vi "SubVI_TurnRight_Auto.vi"(7 "PIDF":dbl[](array[numeric]), 8 "angular Speed":dbl=1000.0, 9 "Degrees to target":dbl) -> ()   [LabVIEW 2017]
uses:
  <vilib>/Rock Robotics/WPI/ThirdParty/Sensors/navX/_TypeDefs/Z900_navX_ActionTypeDef.ctl
  <vilib>/Rock Robotics/WPI/ThirdParty/Sensors/navX/_TypeDefs/FRIC_navX_DeviceNumbersTypeDef.ctl
  <vilib>/Rock Robotics/WPI/ThirdParty/Phoenix-LabVIEW/Motor Controller/Controls/CTRE_Phoenix_MotorControl_ControlMode.ctl
panel:
  out "Yaw":dbl
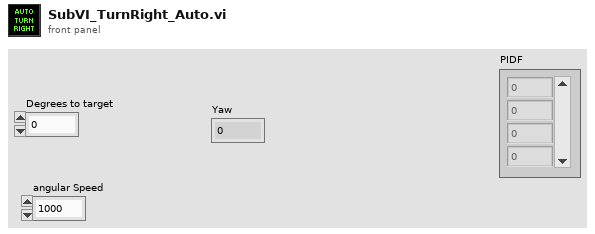
[diagram p1: front panel]
types:
  T1 = typedef "FRIC_navX_DeviceNumbersTypeDef.ctl" = enum16{"Dev0", "Dev1", "Dev2", "Dev3"}
  T2 = typedef "Z900_navX_ActionTypeDef.ctl" = enum16{"None", "Halt", "Normal Read", "Update Serial Protocol", "Update Rate Htz", "Zero-Yaw", "Zero-Displacement", "Zero-Velocity"}
  T3 = typedef "WPI_MotorControlDeviceRef.ctl" = cluster{"DeviceStatus":errorcluster, "Type":T4, "PWM":cluster{"PWM Channel":T5, "DeadBand":T6}, "CAN":cluster{"Device Number":u8, "SetOutput VI Ref":variant, "GetOutput VI Ref":variant, "Enable VI Ref":variant, "Disable VI Ref":variant, "Data":variant}, "Invert":bool, "DIO PWM":cluster{"PWM \"Enable\" Channel":T5, "DIOChannel":T7, "PWM Rate":dbl}}
  T4 = typedef "WPI_MotorControlType.ctl" = enum16{"PWM", "CAN", "DIO PWM"}
  T5 = typedef "FPGA_DIOPWMChannel.ctl" = enum8{"PWM 0", "PWM 1", "PWM 2", "PWM 3", "PWM 4", "PWM 5", "PWM 6", "PWM 7", "PWM 8", "PWM 9", "PWM MXP 0", "PWM MXP 1", "PWM MXP 2", "PWM MXP 3", "PWM MXP 4", "PWM MXP 5", "PWM MXP 6", "PWM MXP 7", "PWM MXP 8", "PWM MXP 9", "Invalid"}
  T6 = typedef "WPI_PWMDeadband.ctl" = cluster{"Name":string, "maxPositivePwm":i32, "minPositivePwm":i32, "centerPwm":i32, "maxNegativePwm":i32, "minNegativePwm":i32, "angularRange":u16}
  T7 = typedef "FPGA_DIOChannel.ctl" = enum8{"DIO 0", "DIO 1", "DIO 2", "DIO 3", "DIO 4", "DIO 5", "DIO 6", "DIO 7", "DIO 8", "DIO 9", "DIO MXP 0", "DIO MXP 1", "DIO MXP 2", "DIO MXP 3", "DIO MXP 4", "DIO MXP 5", "DIO MXP 6", "DIO MXP 7", "DIO MXP 8", "DIO MXP 9", "DIO MXP 10", "DIO MXP 11", "DIO MXP 12", "DIO MXP 13", "DIO MXP 14", "DIO MXP 15", "SPI Port CS1", "SPI Port CS2", "SPI Port CS3", "SPI Port MISO", "SPI Port MOSI", "Invalid"}
  T8 = cluster{"Yaw":dbl, "Roll":dbl, "Pitch":dbl, "Heading":dbl, "Fused Heading":dbl}
  T9 = typedef "CTRE_Phoenix_MotorControl_ControlMode.ctl" = u16
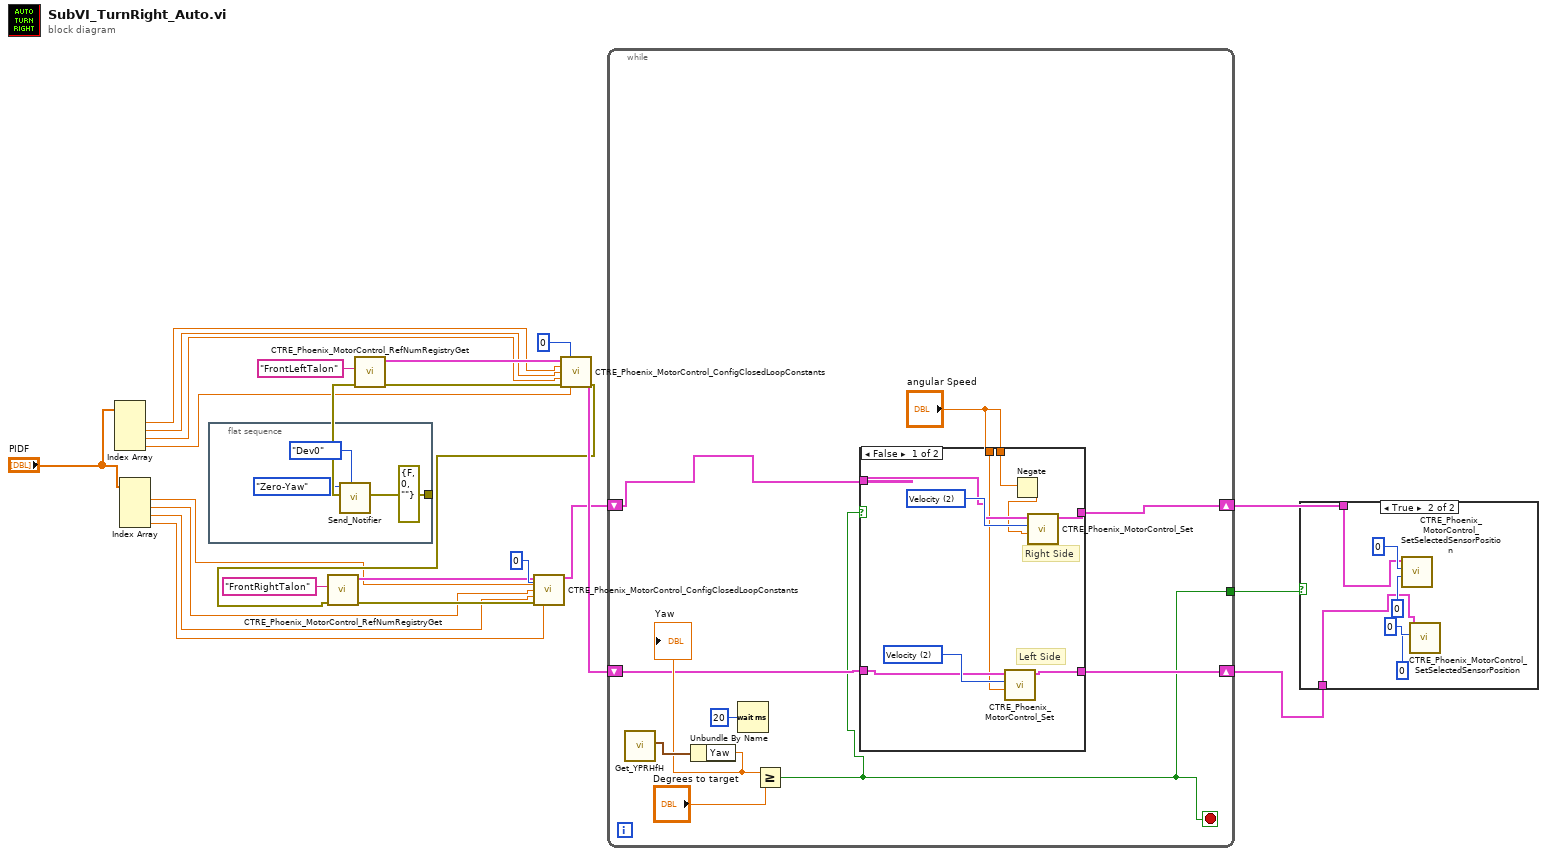
[diagram p0: block diagram]
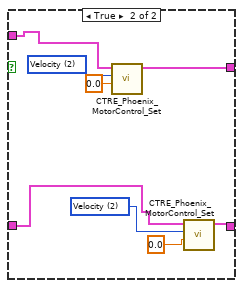
[diagram p3: hidden frame]
diagram:
  n1 = Index Array(array="PIDF") -> (element #1=w11:dbl, element #2=w10:dbl, element #3=w9:dbl, element #4=w8:dbl)  [unwired: 4 in]
  n2 = Index Array(array="PIDF") -> (element #1=w7:dbl, element #2=w6:dbl, element #3=w5:dbl, element #4=w4:dbl)  [unwired: 4 in]
  n3 = flat-sequence {
    tunnel: [errorcluster {"status"=FALSE, "code"=0, "source"=""} ("error constant")] -> w13
    frame #0 {
      n4 = call <vilib>:"Send_Notifier.vi"("Device Number"=FRIC_navX_DeviceNumbersTypeDef."Dev0", "navX Action"=Z900_navX_ActionTypeDef."Zero-Yaw") -> ()  [unwired: 10 in]
    }
  }
  n5 = call <vilib>:"CTRE_Phoenix_MotorControl_RefNumRegistryGet.vi"("error in (no error)"=w13, "refnum name"="FrontLeftTalon") -> ("error out"=w17:errorcluster, "PhoenixMotorControlDevRef"=w18:T3)  [unwired: 8 in]
  n6 = call <vilib>:"CTRE_Phoenix_MotorControl_ConfigClosedLoopConstants.vi"("PhoenixMotorControlDevRef"=w18, "slotIdx"=0, "P"=w11, "I"=w10, "D"=w9, "error in (no error)"=w17, "F"=w8) -> ("PhoenixMotorControlDevRef"=w23:T3, "error out"=w14:errorcluster)  [unwired: 7 in]
  n7 = call <vilib>:"CTRE_Phoenix_MotorControl_RefNumRegistryGet.vi"("error in (no error)"=w14, "refnum name"="FrontRightTalon") -> ("error out"=w15:errorcluster, "PhoenixMotorControlDevRef"=w16:T3)  [unwired: 8 in]
  n8 = call <vilib>:"CTRE_Phoenix_MotorControl_ConfigClosedLoopConstants.vi"("PhoenixMotorControlDevRef"=w16, "slotIdx"=0, "P"=w7, "I"=w6, "D"=w5, "error in (no error)"=w15, "F"=w4) -> ("PhoenixMotorControlDevRef"=w19:T3)  [unwired: 7 in, 1 out]
  n9 = while {
    shift-right: [w31] -> w2
    shift-left: w23 -> [w32]
    shift-right: [w37] -> w3
    shift-left: w19 -> [w35]
    tunnel: [w28] -> w1
    stop <- w28 stop-if-true
    n10 = call <vilib>:"Get_YPRHfH.vi"() -> ("YRPHfH"=w34:T8)  [unwired: 11 in]
    n11 = Unbundle By Name(w34) -> ("Yaw"=w33:dbl)
    "Yaw" <- w33
    n12 = Wait (ms)(milliseconds to wait=u32 20) -> ()  [unwired: 1 out]
    n13 = Greater Or Equal?(x=w33, y="Degrees to target") -> (x >= y?=w28:bool)
    n14 = case shown="False" w28 {
      tunnel: [w45 w52] -> w37
      tunnel: w35 -> [w44 w51]
      tunnel: w32 -> [w42 w49]
      tunnel: [w41 w47] -> w31
      tunnel: "angular Speed" -> [w39 _]
      tunnel: "angular Speed" -> [w40 _]
      frame False {
        w43 = T9 2 items=["PercentOutput"=0, "Position"=1, "Velocity"=2, "Current"=3, "Follower"=5, "MotionProfile"=6, "MotionMagic"=7, "MotionMagicArc"=8, "MotionProfileArc"=10, "Disabled"=15] ("Control Mode")
        w46 = T9 2 items=["PercentOutput"=0, "Position"=1, "Velocity"=2, "Current"=3, "Follower"=5, "MotionProfile"=6, "MotionMagic"=7, "MotionMagicArc"=8, "MotionProfileArc"=10, "Disabled"=15] ("Control Mode")
        # "Right Side"
        # "Left Side"
        n15 = call <vilib>:"CTRE_Phoenix_MotorControl_Set.vi"("Output"=w40, "Control Mode"=w43, "PhoenixMotorControlDevRef"=w42) -> ("PhoenixMotorControlDevRef"=w41:T3)  [unwired: 7 in, 1 out]
        n16 = Negate(x=w39) -> (-x=w38:dbl)
        n17 = call <vilib>:"CTRE_Phoenix_MotorControl_Set.vi"("Output"=w38, "Control Mode"=w46, "PhoenixMotorControlDevRef"=w44) -> ("PhoenixMotorControlDevRef"=w45:T3)  [unwired: 7 in, 1 out]
      }
      frame True {
        w50 = T9 2 items=["PercentOutput"=0, "Position"=1, "Velocity"=2, "Current"=3, "Follower"=5, "MotionProfile"=6, "MotionMagic"=7, "MotionMagicArc"=8, "MotionProfileArc"=10, "Disabled"=15] ("Control Mode")
        w53 = T9 2 items=["PercentOutput"=0, "Position"=1, "Velocity"=2, "Current"=3, "Follower"=5, "MotionProfile"=6, "MotionMagic"=7, "MotionMagicArc"=8, "MotionProfileArc"=10, "Disabled"=15] ("Control Mode")
        n18 = call <vilib>:"CTRE_Phoenix_MotorControl_Set.vi"("Output"=0.0, "Control Mode"=w53, "PhoenixMotorControlDevRef"=w51) -> ("PhoenixMotorControlDevRef"=w52:T3)  [unwired: 7 in, 1 out]
        n19 = call <vilib>:"CTRE_Phoenix_MotorControl_Set.vi"("Output"=0.0, "Control Mode"=w50, "PhoenixMotorControlDevRef"=w49) -> ("PhoenixMotorControlDevRef"=w47:T3)  [unwired: 7 in, 1 out]
      }
    }
  }
  n20 = case shown="True" w1 {
    tunnel: w3 -> [_ w56]
    tunnel: w2 -> [_ w55]
    frame False {
    }
    frame True {
      n21 = call <vilib>:"CTRE_Phoenix_MotorControl_SetSelectedSensorPosition.vi"("pidLoopIdx"=0 ("New Sensor Position"), "New Sensor Position"=u32 0 ("pidLoopIdx"), "PhoenixMotorControlDevRef"=w56) -> ()  [unwired: 7 in, 2 out]
      n22 = call <vilib>:"CTRE_Phoenix_MotorControl_SetSelectedSensorPosition.vi"("pidLoopIdx"=0 ("New Sensor Position"), "New Sensor Position"=u32 0 ("pidLoopIdx"), "PhoenixMotorControlDevRef"=w55) -> ()  [unwired: 7 in, 2 out]
    }
  }
